vi "DriveSetFeet.vi"(1 "Feet":dbl=10.0 format="%#_13g", 3 "Strafe/Move Forward/Backward":T1(ring)) -> (0 "Distance":dbl(knob) scale=0.0..10.0)   [LabVIEW 2014]
panel:
  out "Rate (Rev/Sec)":dbl(knob) scale=0.0..100.0
  in  "Encoder ID":i32
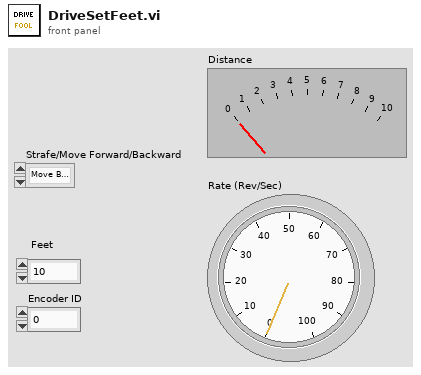
[diagram p1: front panel]
types:
  T1 = enum16{"Move Backward", "Move Forward", "Strafe Right", "Strafe Left"}
  T2 = cluster{"Distance":dbl, "Rate":dbl, "Direction":bool, "Stopped":bool}[]
  T3 = cluster{"Distance":dbl, "Rate":dbl, "Direction":bool, "Stopped":bool}
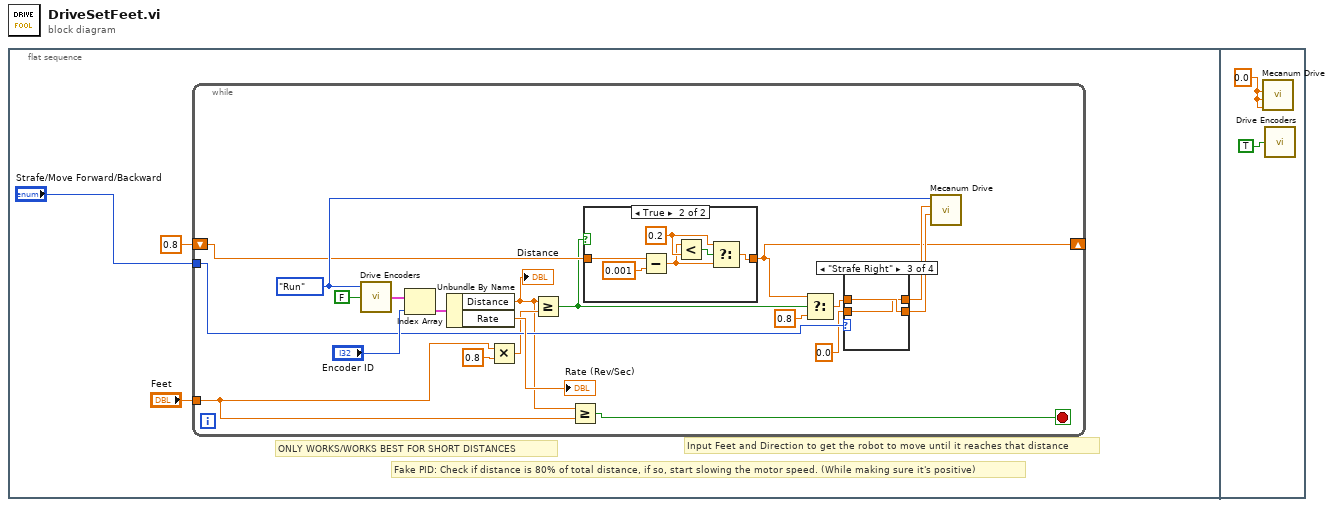
[diagram p0: block diagram]
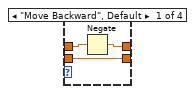
[diagram p3: hidden frame]
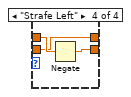
[diagram p5: hidden frame]
diagram:
  n1 = flat-sequence {
    frame #0 {
      # "Input Feet and Direction to get the robot to move until it reaches that distance"
      # "ONLY WORKS/WORKS BEST FOR SHORT DISTANCES"
      # "Fake PID: Check if distance is 80% of total distance, if so, start slowing the motor speed. (While making sure it's positive)"
      n2 = while {
        tunnel: "Strafe/Move Forward/Backward" -> [w17]
        tunnel: "Feet" -> [w12]
        shift-right: [w7] -> _
        shift-left: 0.8 -> [w8]
        stop <- w20 stop-if-true
        w15 = enum8{"Start", "Run", "Finish"}."Run" ("Mode")
        n3 = call "Drive Encoders.vi"("Reset"=FALSE, "Mode"=w15) -> ("Encoder"=w22:T2)  [unwired: 1 in]
        n4 = Index Array(array=w22, index="Encoder ID") -> (element=w21:T3)
        n5 = Unbundle By Name(w21) -> ("Distance"=w6:dbl, "Rate"=→"Rate (Rev/Sec)":dbl)
        "Distance" <- w6
        n6 = Multiply(x=w12, y=0.8) -> (x*y=w10:dbl)
        n7 = Greater Or Equal?(x=w6, y=w10) -> (x >= y?=w5:bool)
        n8 = Greater Or Equal?(x=w6, y=w12) -> (x >= y?=w20:bool)
        n9 = case shown="True" w5 {
          tunnel: w8 -> [w24 w29]
          tunnel: [w24 w25] -> w7
          frame False {
          }
          frame True {
            w27 = 0.2 ("y")
            n10 = Subtract(x=w29, y=0.001) -> (x-y=w26:dbl)
            n11 = Less?(x=w26, y=w27) -> (x < y?=w28:bool)
            n12 = Select(t=w27, s=w28, f=w26) -> (s? t:f=w25:dbl)
          }
        }
        n13 = Select(t=w7, s=w5, f=0.8) -> (s? t:f=w4:dbl)
        n14 = case shown="\"Strafe Right\"" w17 {
          tunnel: w4 -> [w33 w35 w37 w40]
          tunnel: [w32 w35 w36 w38] -> w16
          tunnel: [w31 w34 w37 w39] -> w14
          tunnel: 0.0 ("Turn") -> [w31 w34 w36 w38]
          frame "Move Backward", Default {
            n15 = Negate(x=w33) -> (-x=w32:dbl)
          }
          frame "Move Forward" {
          }
          frame "Strafe Right" {
          }
          frame "Strafe Left" {
            n16 = Negate(x=w40) -> (-x=w39:dbl)
          }
        }
        n17 = call "Mecanum Drive.vi"("Strafe"=w14, "Forward/Backward"=w16, "Mode"=w15) -> ()  [unwired: 9 in]
      }
    }
    frame #1 {
      w42 = 0.0 ("Forward/Backward")
      n18 = call "Mecanum Drive.vi"("Turn"=w42, "Strafe"=w42, "Forward/Backward"=w42) -> ()  [unwired: 9 in]
      n19 = call "Drive Encoders.vi"("Reset"=TRUE) -> ()  [unwired: 2 in, 1 out]
    }
  }
